vi "InitSensor.vi"   [LabVIEW 2019]
uses:
  <vilib>/Rock Robotics/SystemInterfaces/AI/FPGA_AIChannel.ctl
  <vilib>/Rock Robotics/WPI/ThirdParty/Phoenix-LabVIEW/Pigeon IMU/CTRE_PigeonIMU_TareType.ctl
  refnums.vi
  <vilib>/Rock Robotics/WPI/ThirdParty/Phoenix-LabVIEW/Pigeon IMU/CTRE_PigeonIMU_Open_TalonSRX.vi
types:
  T1 = typedef "CTRE_PigeonIMU_TareType.ctl" = u8
  T2 = typedef "FPGA_AIChannel.ctl" = enum8{"AI 0", "AI 1", "AI 2", "AI 3", "AI MXP 0", "AI MXP 1", "AI MXP 2", "AI MXP 3", "Invalid"}
  T3 = typedef "WPI_MotorControlDeviceRef.ctl" = cluster{"DeviceStatus":errorcluster, "Type":T4, "PWM":cluster{"PWM Channel":T5, "DeadBand":T6}, "CAN":cluster{"Device Number":u8, "SetOutput VI Ref":variant, "GetOutput VI Ref":variant, "Enable VI Ref":variant, "Disable VI Ref":variant, "Data":variant}, "Invert":bool, "DIO PWM":cluster{"PWM \"Enable\" Channel":T5, "DIOChannel":T7, "PWM Rate":dbl}}
  T4 = typedef "WPI_MotorControlType.ctl" = enum16{"PWM", "CAN", "DIO PWM"}
  T5 = typedef "FPGA_DIOPWMChannel.ctl" = enum8{"PWM 0", "PWM 1", "PWM 2", "PWM 3", "PWM 4", "PWM 5", "PWM 6", "PWM 7", "PWM 8", "PWM 9", "PWM MXP 0", "PWM MXP 1", "PWM MXP 2", "PWM MXP 3", "PWM MXP 4", "PWM MXP 5", "PWM MXP 6", "PWM MXP 7", "PWM MXP 8", "PWM MXP 9", "Invalid"}
  T6 = typedef "WPI_PWMDeadband.ctl" = cluster{"Name":string, "maxPositivePwm":i32, "minPositivePwm":i32, "centerPwm":i32, "maxNegativePwm":i32, "minNegativePwm":i32, "angularRange":u16}
  T7 = typedef "FPGA_DIOChannel.ctl" = enum8{"DIO 0", "DIO 1", "DIO 2", "DIO 3", "DIO 4", "DIO 5", "DIO 6", "DIO 7", "DIO 8", "DIO 9", "DIO MXP 0", "DIO MXP 1", "DIO MXP 2", "DIO MXP 3", "DIO MXP 4", "DIO MXP 5", "DIO MXP 6", "DIO MXP 7", "DIO MXP 8", "DIO MXP 9", "DIO MXP 10", "DIO MXP 11", "DIO MXP 12", "DIO MXP 13", "DIO MXP 14", "DIO MXP 15", "SPI Port CS1", "SPI Port CS2", "SPI Port CS3", "SPI Port MISO", "SPI Port MOSI", "Invalid"}
  T8 = typedef "CTRE_PigeonIMU_DeviceRef.ctl" = cluster{"DeviceStatus":errorcluster, "Device Number":u8, "Type":T9, "Device ID":u32, "Handle":u64, "UsageFrame":u32, "Library Path":path}
  T9 = typedef "CTRE_PigeonIMU_ConnectionType.ctl" = u32
  T10 = typedef "WPI_PotentiometerDevRef.ctl" = cluster{"DevStatus":errorcluster, "Analog Channel":T2, "Invert Output":bool}
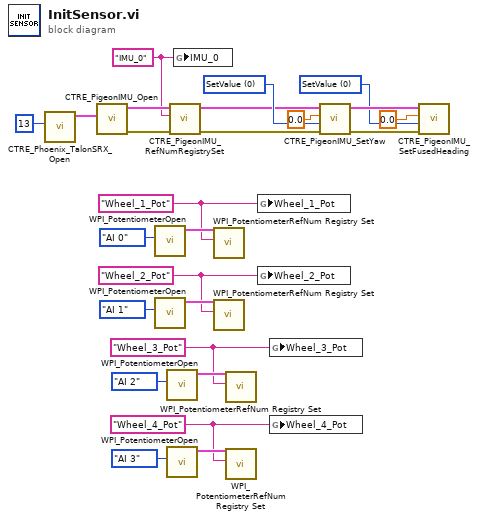
[diagram p0: block diagram]
diagram:
  w10 = T1 0 items=["SetValue"=0, "AddOffset"=1, "MatchCompass"=2, "SetOffset"=255] ("TareType (SetValue)")
  w8 = T1 0 items=["SetValue"=0, "AddOffset"=1, "MatchCompass"=2, "SetOffset"=255] ("TareType (SetValue)")
  w1 = "IMU_0" ("refnum name")
  w14 = "Wheel_4_Pot"
  w17 = "Wheel_3_Pot"
  w20 = "Wheel_2_Pot"
  w23 = "Wheel_1_Pot"
  n1 = call <vilib>:"CTRE_Phoenix_TalonSRX_Open.vi"("Device Number"=u8 13 ("2")) -> ("CAN Talon SRX Ref"=w3:T3)  [unwired: 9 in, 1 out]
  n2 = call-poly <vilib>:"CTRE_PigeonIMU_Open.vi"("CAN Talon SRX Ref"=w3) -> ("error out"=w5:errorcluster, "PigeonIMUDevRef"=w4:T8)  [unwired: 9 in]
  n3 = call <vilib>:"WPI_PotentiometerOpen.vi"("Analog Channel"=FPGA_AIChannel."AI 0") -> ("PotDevRef"=w25:T10)  [unwired: 9 in, 1 out]
  n4 = call <vilib>:"WPI_PotentiometerOpen.vi"("Analog Channel"=FPGA_AIChannel."AI 1") -> ("PotDevRef"=w22:T10)  [unwired: 9 in, 1 out]
  n5 = call <vilib>:"WPI_PotentiometerOpen.vi"("Analog Channel"=FPGA_AIChannel."AI 2") -> ("PotDevRef"=w19:T10)  [unwired: 9 in, 1 out]
  n6 = call <vilib>:"WPI_PotentiometerOpen.vi"("Analog Channel"=FPGA_AIChannel."AI 3") -> ("PotDevRef"=w16:T10)  [unwired: 9 in, 1 out]
  n7 = call <vilib>:"CTRE_PigeonIMU_RefNumRegistrySet.vi"("error in (no error)"=w5, "refnum name"=w1, "PigeonIMUDevRef"=w4) -> ("error out"=w7:errorcluster, "PigeonIMUDevRef"=w6:T8)  [unwired: 7 in]
  n8 = global write "refnums.vi" "IMU_0"(w1) -> ()
  n9 = call <vilib>:"WPI_PotentiometerRefNum Registry Set.vi"("refnum name"=w23, "PotDevRef"=w25) -> ()  [unwired: 8 in, 2 out]
  n10 = call <vilib>:"WPI_PotentiometerRefNum Registry Set.vi"("refnum name"=w20, "PotDevRef"=w22) -> ()  [unwired: 8 in, 2 out]
  n11 = call <vilib>:"WPI_PotentiometerRefNum Registry Set.vi"("refnum name"=w17, "PotDevRef"=w19) -> ()  [unwired: 8 in, 2 out]
  n12 = call <vilib>:"WPI_PotentiometerRefNum Registry Set.vi"("refnum name"=w14, "PotDevRef"=w16) -> ()  [unwired: 8 in, 2 out]
  n13 = global write "refnums.vi" "Wheel_1_Pot"(w23) -> ()
  n14 = global write "refnums.vi" "Wheel_2_Pot"(w20) -> ()
  n15 = global write "refnums.vi" "Wheel_3_Pot"(w17) -> ()
  n16 = global write "refnums.vi" "Wheel_4_Pot"(w14) -> ()
  n17 = call <vilib>:"CTRE_PigeonIMU_SetYaw.vi"("error in (no error)"=w7, "TareType (SetValue)"=w8, "Value"=0.0, "PigeonIMUDevRef"=w6) -> ("error out"=w12:errorcluster, "PigeonIMUDevRef"=w11:T8)  [unwired: 6 in]
  n18 = call <vilib>:"CTRE_PigeonIMU_SetFusedHeading.vi"("error in (no error)"=w12, "TareType (SetValue)"=w10, "Value"=0.0, "PigeonIMUDevRef 2"=w11) -> ()  [unwired: 6 in, 2 out]
